vi "NISE.remote.Connect.vi"(0 "SLSC Remote in":refnum<class "SLSC Interface.lvclass">, 5 "devices":refnum<k21>="$DefaultDevices", 11 "error in (no error)":errorcluster, 12 "connect timeout (60 sec)":dbl=60.0) -> (4 "SLSC Remote out":refnum<class "SLSC Interface.lvclass">, 15 "error out":errorcluster)   [LabVIEW 2016, in "SLSC Interface.lvclass"]
uses:
  SLSC Interface Class/SLSC Interface.lvclass
  SLSC Interface Class/SLSC Interface.lvclass/SLSC Interface.ctl
  SLSC Interface Class/NISE.Read client handle.vi
  SLSC Interface Class/NISE.Read URL.vi
  SLSC Interface Class/NISE.Read session.vi
  <vilib>/httpClient/POSTBuffer.vi
  <vilib>/httpClient/LabVIEWHTTPClient.lvlib
  <vilib>/NI/JSON Support for LabVIEW/JSON Value/JSON Value.lvclass
  <vilib>/NI/NI JSONRPC Server Framework/Classes/Client/JSONRPC Client.lvclass
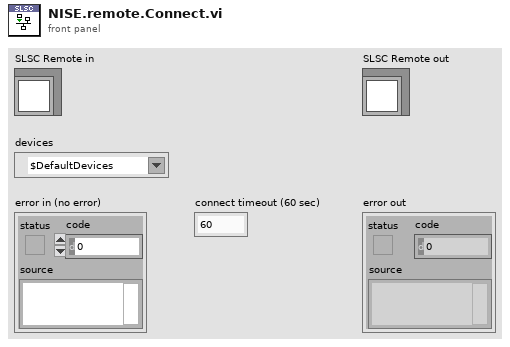
[diagram p1: front panel]
types:
  T1 = typedef "LabVIEWHTTPClient.lvlib/ClientHandle.ctl" = refnum<k1>
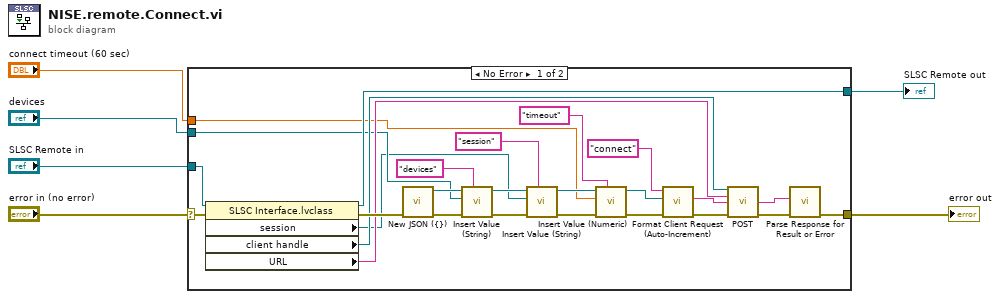
[diagram p0: block diagram]
diagram:
  n1 = case shown="No Error" "error in (no error)" {
    selector: "error in (no error)" -> [w30 w33]
    tunnel: "devices" -> [w8 _]
    tunnel: "SLSC Remote in" -> [w32 w34]
    tunnel: [w31 w34] -> w4
    tunnel: [w19 w33] -> w2
    tunnel: "connect timeout (60 sec)" -> [w9 _]
    frame No Error {
      n2 = property class="SLSC Interface.lvclass"(reference=w32, error in=w30) -> (reference out=w31:refnum<class "SLSC Interface.lvclass">, error out=w29:errorcluster, "session"=w7:refnum<k21>, "client handle"=w24:T1, "URL"=w23:string)
      n3 = call <vilib>:"New JSON ({}).vi"("error in (no error)"=w29) -> ("error out"=w28:errorcluster, "JSON Value out"=w14:refnum<class "JSON Value.lvclass">)  [unwired: 9 in]
      n4 = call <vilib>:"Insert Value (String).vi"("key"="devices" ("Name"), "error in (no error)"=w28, "value"=w8, "JSON Value in"=w14) -> ("error out"=w27:errorcluster, "JSON Value out"=w13:refnum<class "JSON Value.lvclass">)  [unwired: 5 in, 1 out]
      n5 = call <vilib>:"Insert Value (String).vi"("key"="session" ("Name"), "error in (no error)"=w27, "value"=w7, "JSON Value in"=w13) -> ("error out"=w17:errorcluster, "JSON Value out"=w12:refnum<class "JSON Value.lvclass">)  [unwired: 5 in, 1 out]
      n6 = call <vilib>:"Insert Value (Numeric).vi"("key"="timeout" ("Name"), "error in (no error)"=w17, "value"=w9, "JSON Value in"=w12) -> ("error out"=w15:errorcluster, "JSON Value out"=w16:refnum<class "JSON Value.lvclass">)  [unwired: 5 in, 1 out]
      n7 = call <vilib>:"Format Client Request (Auto-Increment).vi"("error in (no error)"=w15, "JSON Value in"=w16, "method"="connect") -> ("error out"=w22:errorcluster, "Request String"=w25:string)  [unwired: 7 in]
      n8 = call-poly <vilib>:"POST.vi"("client handle"=w24, "url"=w23, "buffer"=w25, "error in (no error)"=w22) -> ("body"=w21:string, "error out"=w20:errorcluster)  [unwired: 8 in, 2 out]
      n9 = call <vilib>:"Parse Response for Result or Error.vi"("error in"=w20, "Response String In"=w21) -> ("error out"=w19:errorcluster)  [unwired: 7 in, 2 out]
    }
    frame Error {
    }
  }
  "error out" <- w2
  "SLSC Remote out" <- w4
